vi "Write TestManager.vi"(10 "Test Manager":refnum<class "Basic Test Manager.lvclass">, 11 "Properties in":refnum<class "Properties.lvclass">) -> (3 "Properties out":refnum<class "Properties.lvclass">)   [LabVIEW 2013, in "Caraya.lvlib" / "Properties.lvclass"]
uses:
  Properties.lvclass
  Basic Test Manager/Basic Test Manager.lvclass
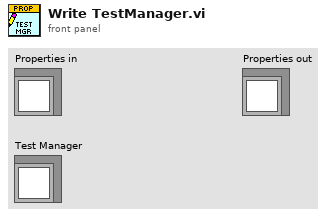
[diagram p1: front panel]
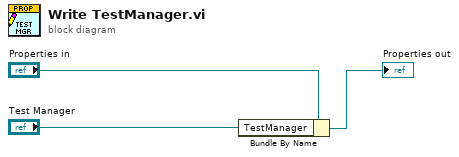
[diagram p0: block diagram]
diagram:
  n1 = Bundle By Name(cluster="Properties in", "TestManager"="Test Manager") -> (→"Properties out":refnum<class "Properties.lvclass">)
